vi "Format String.vi"() -> ()   [LabVIEW 2020]
panel:
  out "Message":string
  in  "Age":u8
  in  "Name":string
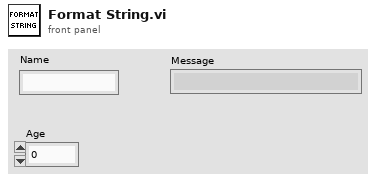
[diagram p1: front panel]
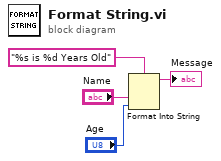
[diagram p0: block diagram]
diagram:
  n1 = Format Into String "Format Into String"(format string="%s is %d Years Old", "Name", "Age") -> (resulting string=→"Message":string)  [unwired: 2 in, 1 out]
